vi "Jump.vi"() -> ()   [LabVIEW 2012]
panel:
  out "元素":string
  out "载入中..请稍候":u8(slide) scale=0.0..100.0
  # "欢迎使用经颅磁治疗仪"
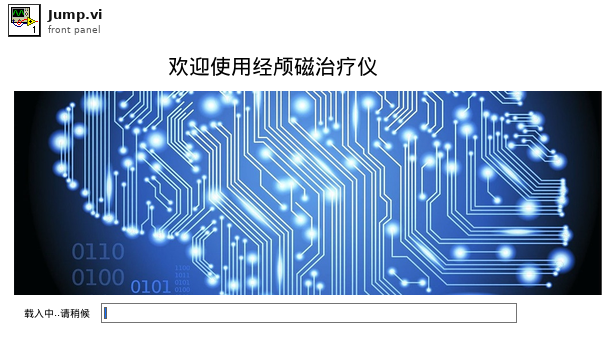
[diagram p1: front panel]
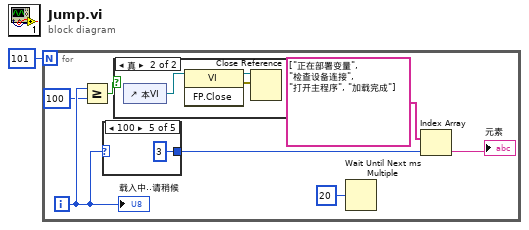
[diagram p0: block diagram]
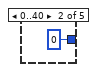
[diagram p4: hidden frame]
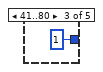
[diagram p5: hidden frame]
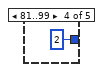
[diagram p6: hidden frame]
diagram:
  n1 = for {
    N: 101 -> [_]
    i -> [w4]
    n2 = Greater Or Equal?(x=w4, y=100) -> (x >= y?=w2:bool)
    n3 = case shown="100" w4 {
      tunnel: [_ 0 1 2 3] -> w6
      frame -1, Default {
      }
      frame 0..40 {
      }
      frame 41..80 {
      }
      frame 81..99 {
      }
      frame 100 {
      }
    }
    n4 = case shown="真" w2 {
      frame False {
      }
      frame True {
        n5 = control-ref of="本VI"() -> (w11:refnum<vi>)
        n6 = invoke class="VI" method="FP.Close"(reference=w11) -> (reference out=w9:refnum<vi>, error out=w10:errorcluster)  [unwired: 2 in, 1 out]
        n7 = Close Reference(reference=w9, error in (no error)=w10) -> ()  [unwired: 1 out]
      }
    }
    n8 = Wait Until Next ms Multiple(millisecond multiple=u32 20 ("毫秒倍数")) -> ()  [unwired: 1 out]
    n9 = Index Array(array=string[] ["正在部署变量", "检查设备连接", "打开主程序", "加载完成"], index=w6) -> (element=→"元素":string)
    "载入中..请稍候" <- w4
  }
